vi "4_4.vi"() -> ()   [LabVIEW 2020]
panel:
  out "Sorted":i64[][](array[numeric])
  in  "Array":i64[][](array[numeric])
  in  "Enum":enum16{"Column", "Row"}(ring)
  in  "Select column":i32 min=0 max=2
  in  "Select row":i32 min=0 max=2
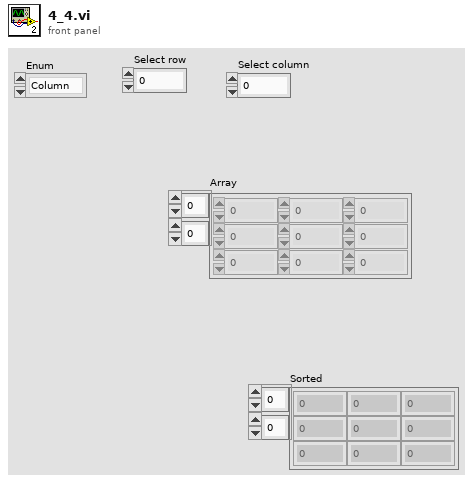
[diagram p1: front panel]
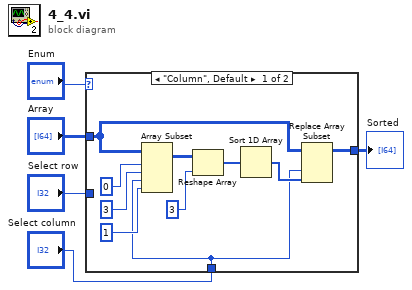
[diagram p0: block diagram]
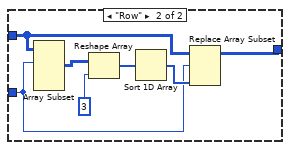
[diagram p2: hidden frame]
diagram:
  n1 = case shown="\"Column\", Default" "Enum" {
    tunnel: "Array" -> [w7 w18]
    tunnel: "Select row" -> [_ w17]
    tunnel: "Select column" -> [w8 _]
    tunnel: [w6 w16] -> w1
    frame "Column", Default {
      n2 = Array Subset(array=w7, index (row)=0 ("index"), length (row)=3 ("length"), index (col)=w8, length (col)=1 ("length")) -> (w14:i64[][])
      n3 = Reshape Array(w14, 3 ("dimension size")) -> (w13:i64[])
      n4 = Sort 1D Array(array=w13) -> (sorted array=w15:i64[])
      n5 = Replace Array Subset(array=w7, new element=w15, index (col)=w8) -> (w6:i64[][])  [unwired: 1 in]
    }
    frame "Row" {
      n6 = Array Subset(array=w18, index (row)=w17) -> (w21:i64[][])  [unwired: 3 in]
      n7 = Reshape Array(w21, 3 ("dimension size")) -> (w20:i64[])
      n8 = Sort 1D Array(array=w20) -> (sorted array=w22:i64[])
      n9 = Replace Array Subset(array=w18, new element=w22, index (row)=w17) -> (w16:i64[][])  [unwired: 1 in]
    }
  }
  "Sorted" <- w1
